vi "Configurations.vi"() -> ()   [LabVIEW 2016]
panel:
  in  "CalibrationsFileLocation":path=path "/home/lvuser/configurations.txt"
  in  "BlueCenterPegDist":dbl=60.0
  in  "BlueOtherDist2":dbl=60.0
  in  "RedOtherDist2":dbl=60.0
  in  "BlueOtherDist1":dbl=80.0
  in  "RedOtherDist1":dbl=80.0
  in  "BlueBoilerDist2":dbl=60.0
  in  "RedBoilerDist2":dbl=60.0
  in  "BlueBoilerDist1":dbl=80.0
  in  "RedBoilerDist1":dbl=80.0
  in  "RedCenterPegDist":dbl=60.0
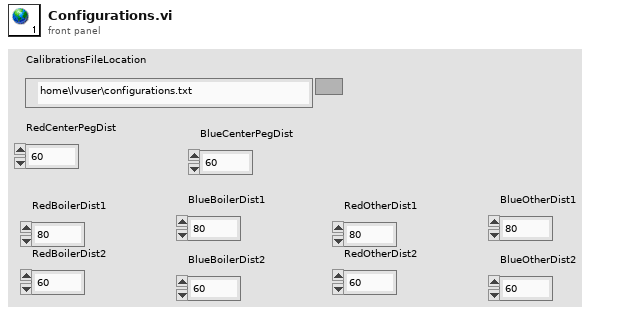
[diagram p1: front panel]
diagram:
